vi "ep_Calculate Symmetrical Components (1 Cycle).vi"(5 "one period fundamental voltage vectors":T2(array[cluster]), 7 "one period fundamental current vectors":T2(array[cluster]), 8 "error in (no error)":errorcluster, 11 "line voltage? (F)":bool) -> (0 "error out":errorcluster, 3 "one-cycle fundamental symmetrical components":T3(array[cluster]))   [LabVIEW 2014, in "NI_EP_Power Quality.lvlib"]
uses:
  <vilib>/addons/Electrical Power/PQ/NI_EP_Power Quality.lvlib
  <vilib>/addons/Electrical Power/PQ/Common/Controls/ep_AI Data Channel.ctl
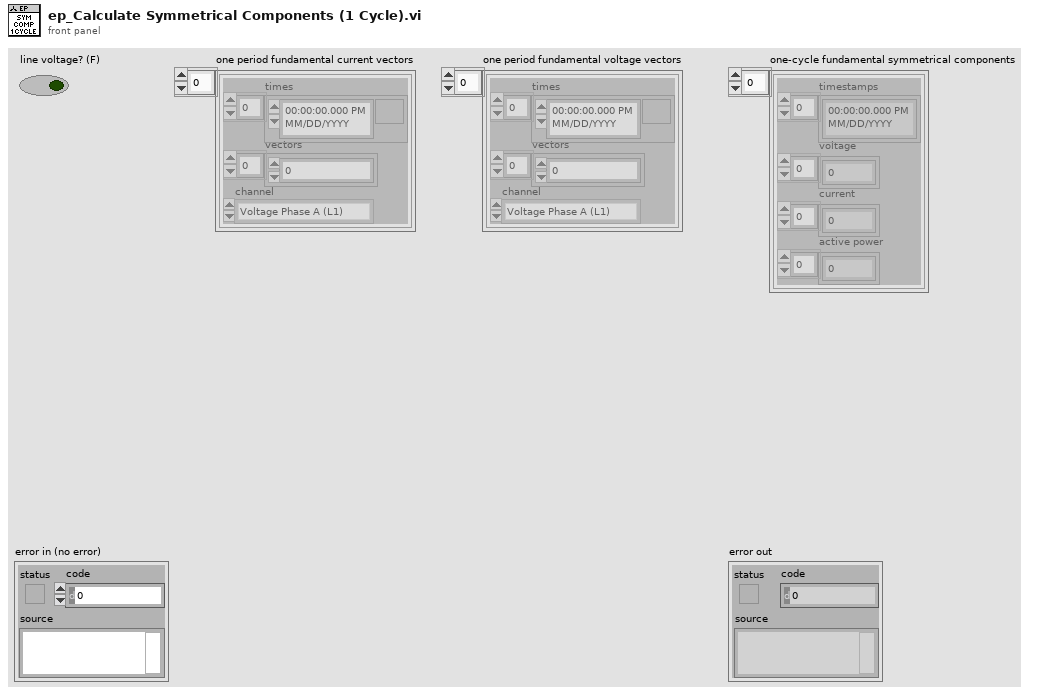
[diagram p1: front panel]
types:
  T1 = typedef "NI_EP_Power Quality.lvlib/ep_AI Data Channel.ctl" = enum16{"Voltage Phase A (L1)", "Voltage Phase B (L2)", "Voltage Phase C (L3)", "Voltage Phase N (Neutral)", "Current Phase A (L1)", "Current Phase B (L2)", "Current Phase C (L3)", "Current Phase N (Neutral)"}
  T2 = cluster{"times":timestamp[], "vectors":cdb[], "channel":T1}[]
  T3 = cluster{"timestamps":timestamp[], "voltage":dbl[], "current":dbl[], "active power":dbl[]}[]
  T4 = cluster{"times":timestamp[], "zero":cdb[], "positive":cdb[], "negative":cdb[]}
  T5 = cluster{"times":timestamp[], dbl[], dbl[], dbl[]}
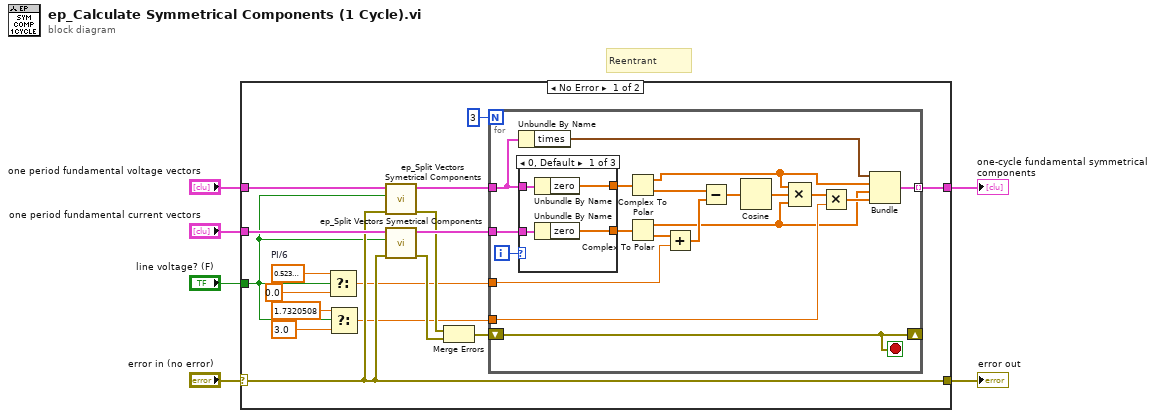
[diagram p0: block diagram]
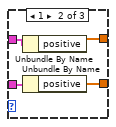
[diagram p2: hidden frame]
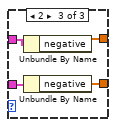
[diagram p3: hidden frame]
diagram:
  # "Reentrant"
  n1 = case shown="No Error" "error in (no error)" {
    selector: "error in (no error)" -> [w14 w55]
    tunnel: "one period fundamental voltage vectors" -> [w20 _]
    tunnel: "one period fundamental current vectors" -> [w19 _]
    tunnel: [w15 _] -> w4
    tunnel: [w14 w55] -> w2
    tunnel: "line voltage? (F)" -> [w7 _]
    frame No Error {
      w12 = 0.5235987755982988  # PI/6
      n2 = Select(t=w12, s=w7, f=0.0) -> (s? t:f=w9:dbl)
      n3 = Select(t=1.7320508 ("x"), s=w7, f=3.0 ("x")) -> (s? t:f=w8:dbl)
      n4 = call <vilib>:"ep_Split Vectors Symetrical Components.vi"("error in (no error)"=w14, "line voltage? (F)"=w7, "one period fundamental vectors"=w20) -> ("error out"=w18:errorcluster, "spectra symetrical components"=w22:T4)  [unwired: 7 in]
      n5 = call <vilib>:"ep_Split Vectors Symetrical Components.vi"("error in (no error)"=w14, "line voltage? (F)"=w7, "one period fundamental vectors"=w19) -> ("error out"=w17:errorcluster, "spectra symetrical components"=w21:T4)  [unwired: 7 in]
      n6 = Merge Errors(w18, w17) -> (w16:errorcluster)
      n7 = for {
        N: 3 -> [_]
        tunnel: w8 -> [w37]
        tunnel: w22 -> [w27]
        tunnel: w21 -> [w36]
        tunnel: [w30] -> w15 mode=indexing
        tunnel: w9 -> [w24]
        shift-right: [w25] -> _
        shift-left: w16 -> [w25]
        i -> [w33]
        stop <- w25 stop-if-true
        n8 = Unbundle By Name(w27) -> ("times"=w26:timestamp[])
        n9 = case shown="0, Default" w33 {
          tunnel: w27 -> [w46 w50 w54]
          tunnel: [w45 w49 w53] -> w35
          tunnel: w36 -> [w44 w48 w52]
          tunnel: [w43 w47 w51] -> w34
          frame 0, Default {
            n10 = Unbundle By Name(w46) -> ("zero"=w45:cdb[])
            n11 = Unbundle By Name(w44) -> ("zero"=w43:cdb[])
          }
          frame 1 {
            n12 = Unbundle By Name(w50) -> ("positive"=w49:cdb[])
            n13 = Unbundle By Name(w48) -> ("positive"=w47:cdb[])
          }
          frame 2 {
            n14 = Unbundle By Name(w54) -> ("negative"=w53:cdb[])
            n15 = Unbundle By Name(w52) -> ("negative"=w51:cdb[])
          }
        }
        n16 = Complex To Polar(r * e^(i*theta)=w35) -> (r=w29:dbl[], theta=w42:dbl[])
        n17 = Complex To Polar(r * e^(i*theta)=w34) -> (r=w28:dbl[], theta=w41:dbl[])
        n18 = Add(x=w41, y=w24) -> (x+y=w40:dbl[])
        n19 = Subtract(x=w42, y=w40) -> (x-y=w38:dbl[])
        n20 = Cosine(x=w38) -> (cos(x)=w39:dbl[])
        n21 = Compound Arithmetic op=MULTIPLY(w29, w39, w28) -> (w32:dbl[])
        n22 = Multiply(x=w32, y=w37) -> (x*y=w31:dbl[])
        n23 = Bundle("times"=w26, w29, w28, w31) -> (w30:T5)  [unwired: 1 in]
      }
    }
    frame Error {
    }
  }
  "one-cycle fundamental symmetrical components" <- w4
  "error out" <- w2
